vi "F Dwf Digital IO Output Enable Get64.vi"(8 "error in (no error)":errorcluster, 10 "pfsOutputEnable":cluster{}, 11 "hdwf":i32) -> (0 "error out":errorcluster, 2 "pfsOutputEnable out":cluster{}, 3 "function return":i32)   [LabVIEW 2019, in "Olasdwf.lvlib"]
doc: "DWFAPI int FDwfDigitalIOOutputEnableGet64(HDWF hdwf, unsigned long long *pfsOutputEnable);"
uses:
  Olasdwf.lvlib
  Windows/System32/dwf.dll
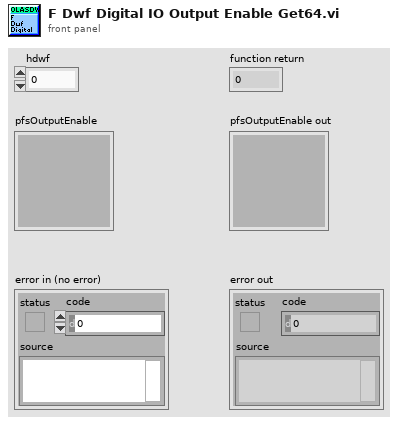
[diagram p1: front panel]
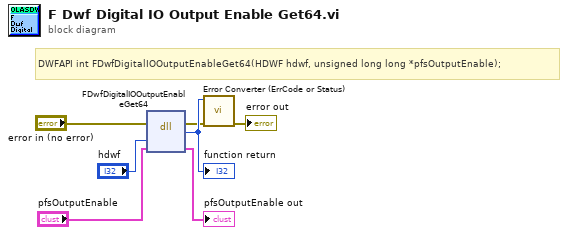
[diagram p0: block diagram]
diagram:
  # "DWFAPI int FDwfDigitalIOOutputEnableGet64(HDWF hdwf, unsigned long long *pfsOutputEnable);"
  n1 = dll-call lib="C:/Windows/System32/dwf.*" fn="FDwfDigitalIOOutputEnableGet64"(error in="error in (no error)", "hdwf"="hdwf", "pfsOutputEnable"="pfsOutputEnable") -> (error out=w2:errorcluster, w7:i32, "pfsOutputEnable"=→"pfsOutputEnable out":cluster{})  [unwired: 3 in, 1 out]
  "function return" <- w7
  n2 = call "Error Converter (ErrCode or Status).vi"("error in (no error)"=w2, "error code"=w7) -> ("error out"=→"error out":errorcluster)  [unwired: 9 in]
